vi "Send Set Output Range.vi"(8 "error in (no error)":errorcluster, 10 "output range":cluster{"output high":dbl, "output low":dbl}={"output high"=100.0, "output low"=-100.0} {"output low" format="%.2f"; "output high" format="%.2f"}, 11 "Message Queue in":refnum<queue>) -> (0 "error out":errorcluster, 3 "Message Queue out":refnum<queue>)   [LabVIEW 2024, in "PID Loop.lvlib" / "Set Output Range.lvclass"]
uses:
  Set Output Range.lvclass
  Set Output Range.lvclass/Set Output Range.ctl
  C:/Users/uspoaotto/OneDrive - Oregon Tool/Desktop/working copies/helperLoop/src/OOQMH/Message/Message.lvclass
  C:/Users/uspoaotto/OneDrive - Oregon Tool/Desktop/working copies/helperLoop/src/PID Loop/Set Output Range/Set Output Range.lvclass
  OOQMH/Message/Message.lvclass
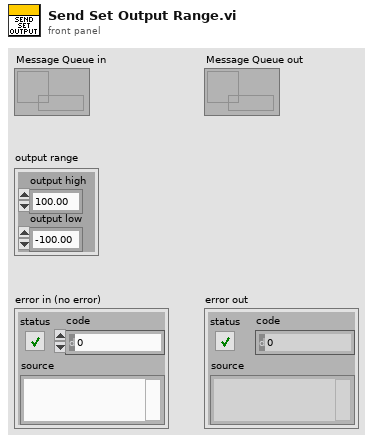
[diagram p1: front panel]
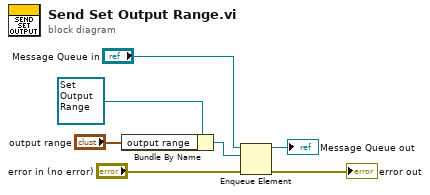
[diagram p0: block diagram]
diagram:
  n1 = Bundle By Name(cluster=refnum<class "Set Output Range.lvclass"> refnum ("PID Loop.lvlib:Set Output Range.lvclass"), "output range"="output range") -> (w4:refnum<class "Set Output Range.lvclass">)
  n2 = Enqueue Element(queue="Message Queue in", element=w4, error in (no error)="error in (no error)") -> (queue out=→"Message Queue out":refnum<queue>, error out=→"error out":errorcluster)  [unwired: 1 in, 1 out]
